vi "FGV Modules References.vi"(7 "size(s)":i32, 9 "Module_Refs":T1={"ModuleName"=enum."Controller", "Queue"=refnum, "user event"=refnum, "VI Refnum"=refnum, "ShowFP"=FALSE, "StatesTracking Enabled"=FALSE}, 10 "App Module Ref":refnum<vi>, 11 "FGV Ref. Function In":T3) -> (0 "error out":errorcluster, 1 "Module_Ref Out":T1={"ModuleName"=enum."Controller", "Queue"=refnum, "user event"=refnum, "VI Refnum"=refnum, "ShowFP"=FALSE, "StatesTracking Enabled"=FALSE}, 3 "All Modules Refs":T1[](array[typedef]), 5 "size out":i32)   [LabVIEW 2021, in "Architecture.lvlib"]
doc: "This FGV stores all references from all modules to be used all around the application to access them. \n\nInit: Use it on application startup. \nAdd: Use it once a new module is initialized in the application to store the references of it. \nGet: Pass a module name to search its references and return them on \"Module_Ref Out\" output. \nGet All: returns all references on \"All modules refs.\"\nDispose: Use it to close all references for all modules. To be used on application stop sequence."
uses:
  Architecture.lvlib
  Typedefs/FGV Ref. Modules Function.ctl
  Typedefs/Module References.ctl
  Typedefs/Enum_Module_Name.ctl
  Typedefs/Message.ctl
  Modules/Configuration/Configuration.lvlib
panel:
  in  "error in":errorcluster
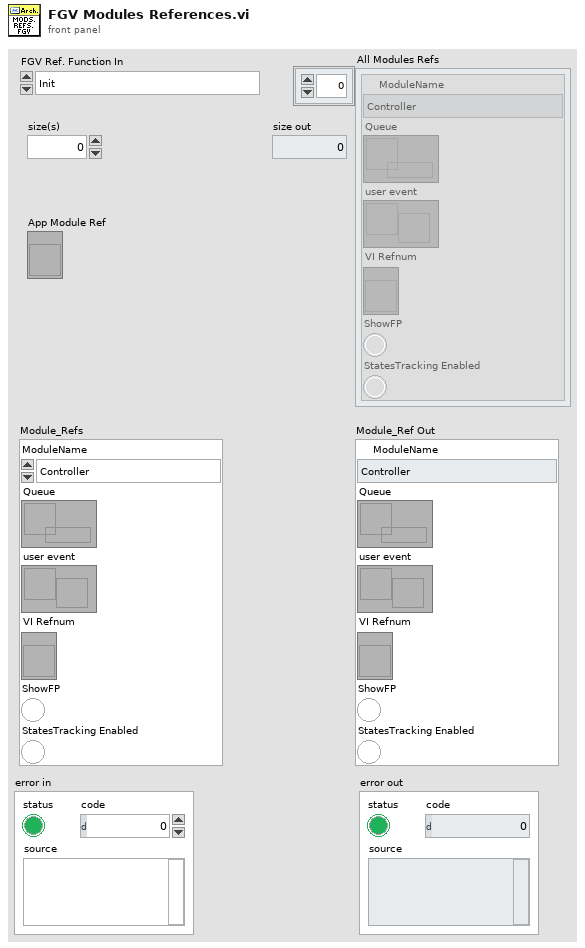
[diagram p1: front panel]
types:
  T1 = typedef "Architecture.lvlib/Module References.ctl" = cluster{"ModuleName":T2, "Queue":refnum<queue>, "user event":refnum<user-event>, "VI Refnum":refnum<vi>, "ShowFP":bool, "StatesTracking Enabled":bool}
  T2 = typedef "Configuration.lvlib/Enum_Module_Name.ctl" = enum16{"Configuration", "Error_Handler", "Log", "Database", "Controller"}
  T3 = typedef "Architecture.lvlib/FGV Ref. Modules Function.ctl" = enum16{"Init ", "Add Module", "Get Module", "Get All", "Add Asynchronous Run Ref", "Dispose"}
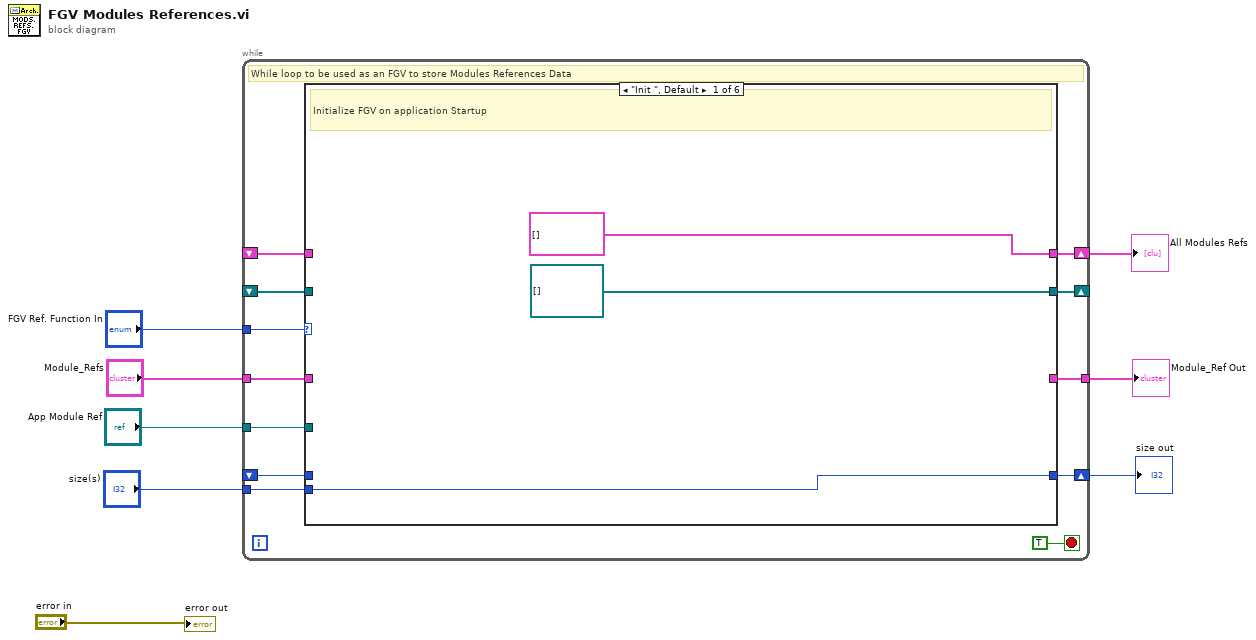
[diagram p0: block diagram]
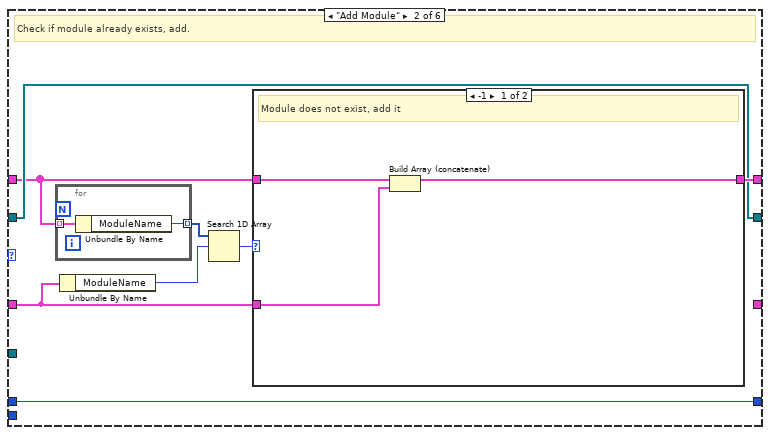
[diagram p2: hidden frame]
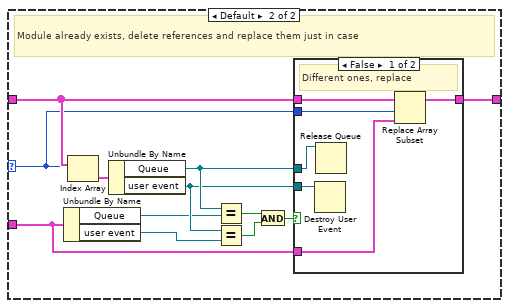
[diagram p3: hidden frame]
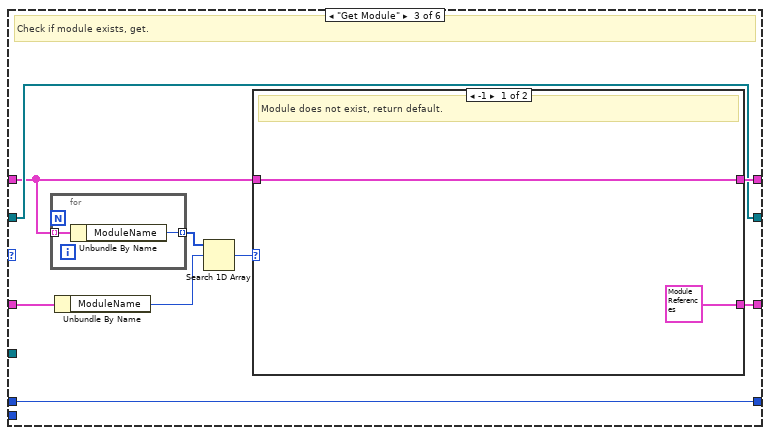
[diagram p5: hidden frame]
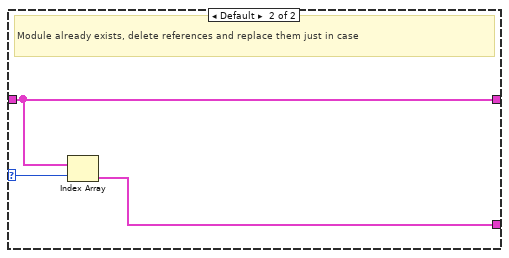
[diagram p6: hidden frame]
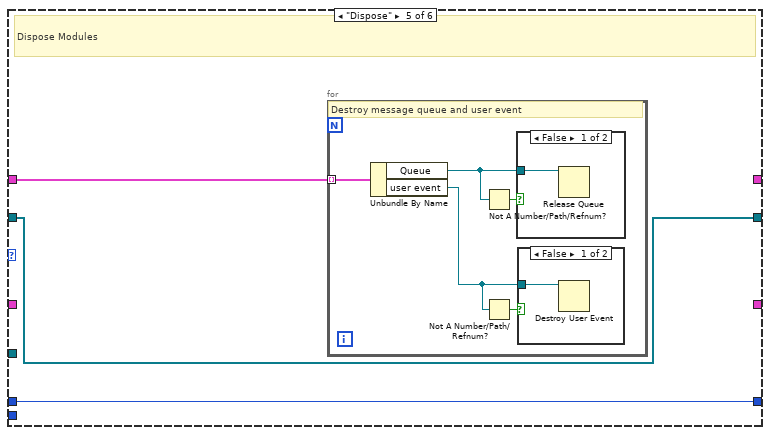
[diagram p8: hidden frame]
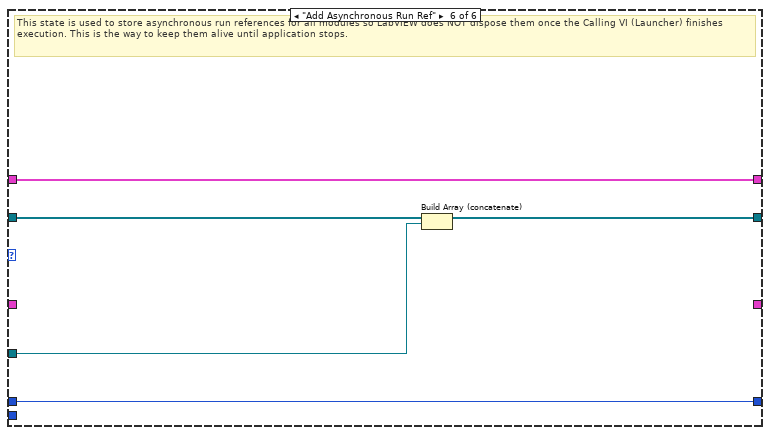
[diagram p11: hidden frame]
diagram:
  n1 = while {
    tunnel: "FGV Ref. Function In" -> [w19]
    shift-right: [w18] -> w5
    shift-left: _ -> [w17]
    tunnel: "Module_Refs" -> [w16]
    tunnel: [w15] -> w6
    tunnel: "App Module Ref" -> [w14]
    shift-right: [w13] -> _
    shift-left: _ -> [w12]
    shift-right: [w10] -> w2
    shift-left: _ -> [w11]
    tunnel: "size(s)" -> [w9]
    stop <- TRUE stop-if-true
    # "While loop to be used as an FGV to store Modules References Data"
    n2 = case shown="\"Init \", Default" w19 {
      tunnel: [T1[] [] w31 w63 w74 _ w86] -> w18
      tunnel: w17 -> [_ w26 w58 w74 w77 w86]
      tunnel: w16 -> [_ w28 w62 _ _ _]
      tunnel: [_ _ w61 _ _ _] -> w15
      tunnel: w14 -> [_ _ _ _ _ w87]
      tunnel: [refnum<vi>[] [] ("App Module Ref") w30 w60 w73 w76 w88] -> w13
      tunnel: w12 -> [_ w30 w60 w73 w76 w89]
      tunnel: w11 -> [_ w24 w56 w72 w75 w85]
      tunnel: [w21 w24 w56 w72 w75 w85] -> w10
      tunnel: w9 -> [w21 _ _ _ _ _]
      frame "Init ", Default {
        # "Initialize FGV on application Startup"
      }
      frame "Add Module" {
        # "Check if module already exists, add."
        n3 = for {
          tunnel: w26 -> [w33] mode=indexing
          tunnel: [w32] -> w29 mode=indexing
          n4 = Unbundle By Name(w33) -> ("ModuleName"=w32:T2)
        }
        n5 = Unbundle By Name(w28) -> ("ModuleName"=w27:T2)
        n6 = Search 1D Array(1D array=w29, element=w27) -> (index of element=w25:i32)  [unwired: 1 in]
        n7 = case shown="-1" w25 {
          selector: w25 -> [_ w38]
          tunnel: w26 -> [w36 w48]
          tunnel: [w35 w46] -> w31
          tunnel: w28 -> [w34 w37]
          frame -1 {
            # "Module does not exist, add it"
            n8 = Build Array (concatenate)(w36, w34) -> (w35:T1[])
          }
          frame Default {
            # "Module already exists, delete references and replace them just in case"
            n9 = Unbundle By Name(w37) -> ("Queue"=w43:refnum<queue>, "user event"=w42:refnum<user-event>)
            n10 = Index Array(array=w48, index=w38) -> (element=w47:T1)
            n11 = Unbundle By Name(w47) -> ("Queue"=w45:refnum<queue>, "user event"=w44:refnum<user-event>)
            n12 = Equal?(x=w45, y=w43) -> (x = y?=w41:bool)
            n13 = Equal?(x=w44, y=w42) -> (x = y?=w40:bool)
            n14 = And(x=w41, y=w40) -> (x .and. y?=w39:bool)
            n15 = case shown="False" w39 {
              tunnel: w48 -> [w54 w55]
              tunnel: [w53 w55] -> w46
              tunnel: w45 -> [w52 _]
              tunnel: w44 -> [w51 _]
              tunnel: w38 -> [w50 _]
              tunnel: w37 -> [w49 _]
              frame False {
                # "Different ones, replace"
                n16 = Destroy User Event(user event=w51) -> ()  [unwired: 1 in, 1 out]
                n17 = Release Queue(queue=w52) -> ()  [unwired: 2 in, 3 out]
                n18 = Replace Array Subset(array=w54, new element=w49, index=w50) -> (w53:T1[])
              }
              frame True {
                # "Same refs, do nothing"
              }
            }
          }
        }
      }
      frame "Get Module" {
        # "Check if module exists, get."
        n19 = for {
          tunnel: w58 -> [w66] mode=indexing
          tunnel: [w65] -> w57 mode=indexing
          n20 = Unbundle By Name(w66) -> ("ModuleName"=w65:T2)
        }
        n21 = Unbundle By Name(w62) -> ("ModuleName"=w59:T2)
        n22 = Search 1D Array(1D array=w57, element=w59) -> (index of element=w64:i32)  [unwired: 1 in]
        n23 = case shown="-1" w64 {
          selector: w64 -> [_ w70]
          tunnel: w58 -> [w68 w71]
          tunnel: [w68 w71] -> w63
          tunnel: [T1 {"ModuleName"=enum."Controller", "Queue"=refnum, "user event"=refnum, "VI Refnum"=refnum, "ShowFP"=FALSE, "StatesTracking Enabled"=FALSE} ("Module_Ref Out") w69] -> w61
          frame -1 {
            # "Module does not exist, return default."
          }
          frame Default {
            # "Module already exists, delete references and replace them just in case"
            n24 = Index Array(array=w71, index=w70) -> (element=w69:T1)
          }
        }
      }
      frame "Get All" {
        # "Return all modules"
      }
      frame "Dispose" {
        # "Dispose Modules"
        n25 = for {
          tunnel: w77 -> [w82] mode=indexing
          # "Destroy message queue and user event"
          n26 = Unbundle By Name(w82) -> ("Queue"=w81:refnum<queue>, "user event"=w79:refnum<user-event>)
          n27 = Not A Number/Path/Refnum?(number/path/refnum=w81) -> (NaN/Path/Refnum?=w80:bool)
          n28 = Not A Number/Path/Refnum?(number/path/refnum=w79) -> (NaN/Path/Refnum?=w78:bool)
          n29 = case shown="False" w80 {
            tunnel: w81 -> [w84 _]
            frame False {
              n30 = Release Queue(queue=w84) -> ()  [unwired: 2 in, 3 out]
            }
            frame True {
            }
          }
          n31 = case shown="False" w78 {
            tunnel: w79 -> [w83 _]
            frame False {
              n32 = Destroy User Event(user event=w83) -> ()  [unwired: 1 in, 1 out]
            }
            frame True {
            }
          }
        }
      }
      frame "Add Asynchronous Run Ref" {
        # "This state is used to store asynchronous run references for all modules so LabVIEW does NOT dispose them once the Calling VI (Launcher) finishes execution. This is the way to keep them alive until application stops."
        n33 = Build Array (concatenate)(w89, w87) -> (w88:refnum<vi>[])
      }
    }
  }
  "Module_Ref Out" <- w6
  "All Modules Refs" <- w5
  "size out" <- w2
  "error out" <- "error in"
